vi "USB2CANFD_SchTest.vi"() -> ()   [LabVIEW 2010]
panel:
  in  "SpeedBpsDBT":u32(ring)=2000000 items=["5000 Kbps"=5000000, "2000 Kbps"=2000000, "1000 Kbps"=1000000, "500 Kbps"=500000, "250 Kbps"=250000, "200 Kbps"=200000, "125 Kbps"=125000, "100 Kbps"=100000, ""=0]
  in  "SpeedBpsNBT":u32(ring)=500000 items=["1000 Kbps"=1000000, "500 Kbps"=500000, "250 Kbps"=250000, "200 Kbps"=200000, "125 Kbps"=125000, "100 Kbps"=100000, ""=0]
  in  "TimePrecMs":u8=10
  in  "MsgTabIndex":u8
  in  "CanSendMsg7":T1={"ID"=7, "DLC"=8, "Flags"=0, "__Res0"=0, "__Res1"=0, "TimeStamp"=20, "Data[0]"=1, "Data[1]"=2, "Data[2]"=3, "Data[3]"=4, "Data[4]"=5, "Data[5]"=6, "Data[6]"=7, "Data[7]"=8, "Data[8]"=0, "Data[9]"=0, "Data[10]"=0, "Data[11]"=0, "Data[12]"=0, "Data[13]"=0, "Data[14]"=0, "Data[15]"=0, "Data[16]"=0, "Data[17]"=0, "Data[18]"=0, "Data[19]"=0, "Data[20]"=0, "Data[21]"=0, "Data[22]"=0, "Data[23]"=0, "Data[24]"=0, "Data[25]"=0, "Data[26]"=0, "Data[27]"=0, "Data[28]"=0, "Data[29]"=0, "Data[30]"=0, "Data[31]"=0, "Data[32]"=0, "Data[33]"=0, "Data[34]"=0, "Data[35]"=0, "Data[36]"=0, "Data[37]"=0, "Data[38]"=0, "Data[39]"=0, "Data[40]"=0, "Data[41]"=0, "Data[42]"=0, "Data[43]"=0, "Data[44]"=0, "Data[45]"=0, "Data[46]"=0, "Data[47]"=0, "Data[48]"=0, "Data[49]"=0, "Data[50]"=0, "Data[51]"=0, "Data[52]"=0, "Data[53]"=0, "Data[54]"=0, "Data[55]"=0, "Data[56]"=0, "Data[57]"=0, "Data[58]"=0, "Data[59]"=0, "Data[60]"=0, "Data[61]"=0, "Data[62]"=0, "Data[63]"=0} {"ID" format="%x"; "Data[1]" format="%x"; "Data[2]" format="%x"}
  in  "CanSendMsg6":T1={"ID"=6, "DLC"=8, "Flags"=0, "__Res0"=0, "__Res1"=0, "TimeStamp"=20, "Data[0]"=1, "Data[1]"=2, "Data[2]"=3, "Data[3]"=4, "Data[4]"=5, "Data[5]"=6, "Data[6]"=7, "Data[7]"=8, "Data[8]"=0, "Data[9]"=0, "Data[10]"=0, "Data[11]"=0, "Data[12]"=0, "Data[13]"=0, "Data[14]"=0, "Data[15]"=0, "Data[16]"=0, "Data[17]"=0, "Data[18]"=0, "Data[19]"=0, "Data[20]"=0, "Data[21]"=0, "Data[22]"=0, "Data[23]"=0, "Data[24]"=0, "Data[25]"=0, "Data[26]"=0, "Data[27]"=0, "Data[28]"=0, "Data[29]"=0, "Data[30]"=0, "Data[31]"=0, "Data[32]"=0, "Data[33]"=0, "Data[34]"=0, "Data[35]"=0, "Data[36]"=0, "Data[37]"=0, "Data[38]"=0, "Data[39]"=0, "Data[40]"=0, "Data[41]"=0, "Data[42]"=0, "Data[43]"=0, "Data[44]"=0, "Data[45]"=0, "Data[46]"=0, "Data[47]"=0, "Data[48]"=0, "Data[49]"=0, "Data[50]"=0, "Data[51]"=0, "Data[52]"=0, "Data[53]"=0, "Data[54]"=0, "Data[55]"=0, "Data[56]"=0, "Data[57]"=0, "Data[58]"=0, "Data[59]"=0, "Data[60]"=0, "Data[61]"=0, "Data[62]"=0, "Data[63]"=0} {"ID" format="%x"; "Data[1]" format="%x"; "Data[2]" format="%x"}
  in  "CanSendMsg5":T1={"ID"=5, "DLC"=8, "Flags"=0, "__Res0"=0, "__Res1"=0, "TimeStamp"=20, "Data[0]"=1, "Data[1]"=2, "Data[2]"=3, "Data[3]"=4, "Data[4]"=5, "Data[5]"=6, "Data[6]"=7, "Data[7]"=8, "Data[8]"=0, "Data[9]"=0, "Data[10]"=0, "Data[11]"=0, "Data[12]"=0, "Data[13]"=0, "Data[14]"=0, "Data[15]"=0, "Data[16]"=0, "Data[17]"=0, "Data[18]"=0, "Data[19]"=0, "Data[20]"=0, "Data[21]"=0, "Data[22]"=0, "Data[23]"=0, "Data[24]"=0, "Data[25]"=0, "Data[26]"=0, "Data[27]"=0, "Data[28]"=0, "Data[29]"=0, "Data[30]"=0, "Data[31]"=0, "Data[32]"=0, "Data[33]"=0, "Data[34]"=0, "Data[35]"=0, "Data[36]"=0, "Data[37]"=0, "Data[38]"=0, "Data[39]"=0, "Data[40]"=0, "Data[41]"=0, "Data[42]"=0, "Data[43]"=0, "Data[44]"=0, "Data[45]"=0, "Data[46]"=0, "Data[47]"=0, "Data[48]"=0, "Data[49]"=0, "Data[50]"=0, "Data[51]"=0, "Data[52]"=0, "Data[53]"=0, "Data[54]"=0, "Data[55]"=0, "Data[56]"=0, "Data[57]"=0, "Data[58]"=0, "Data[59]"=0, "Data[60]"=0, "Data[61]"=0, "Data[62]"=0, "Data[63]"=0} {"ID" format="%x"; "Data[1]" format="%x"; "Data[2]" format="%x"}
  in  "CanSendMsg4":T1={"ID"=4, "DLC"=8, "Flags"=0, "__Res0"=0, "__Res1"=0, "TimeStamp"=20, "Data[0]"=1, "Data[1]"=2, "Data[2]"=3, "Data[3]"=4, "Data[4]"=5, "Data[5]"=6, "Data[6]"=7, "Data[7]"=8, "Data[8]"=0, "Data[9]"=0, "Data[10]"=0, "Data[11]"=0, "Data[12]"=0, "Data[13]"=0, "Data[14]"=0, "Data[15]"=0, "Data[16]"=0, "Data[17]"=0, "Data[18]"=0, "Data[19]"=0, "Data[20]"=0, "Data[21]"=0, "Data[22]"=0, "Data[23]"=0, "Data[24]"=0, "Data[25]"=0, "Data[26]"=0, "Data[27]"=0, "Data[28]"=0, "Data[29]"=0, "Data[30]"=0, "Data[31]"=0, "Data[32]"=0, "Data[33]"=0, "Data[34]"=0, "Data[35]"=0, "Data[36]"=0, "Data[37]"=0, "Data[38]"=0, "Data[39]"=0, "Data[40]"=0, "Data[41]"=0, "Data[42]"=0, "Data[43]"=0, "Data[44]"=0, "Data[45]"=0, "Data[46]"=0, "Data[47]"=0, "Data[48]"=0, "Data[49]"=0, "Data[50]"=0, "Data[51]"=0, "Data[52]"=0, "Data[53]"=0, "Data[54]"=0, "Data[55]"=0, "Data[56]"=0, "Data[57]"=0, "Data[58]"=0, "Data[59]"=0, "Data[60]"=0, "Data[61]"=0, "Data[62]"=0, "Data[63]"=0} {"ID" format="%x"; "Data[1]" format="%x"; "Data[2]" format="%x"}
  in  "CanSendMsg3":T1={"ID"=3, "DLC"=8, "Flags"=0, "__Res0"=0, "__Res1"=0, "TimeStamp"=20, "Data[0]"=1, "Data[1]"=2, "Data[2]"=3, "Data[3]"=4, "Data[4]"=5, "Data[5]"=6, "Data[6]"=7, "Data[7]"=8, "Data[8]"=0, "Data[9]"=0, "Data[10]"=0, "Data[11]"=0, "Data[12]"=0, "Data[13]"=0, "Data[14]"=0, "Data[15]"=0, "Data[16]"=0, "Data[17]"=0, "Data[18]"=0, "Data[19]"=0, "Data[20]"=0, "Data[21]"=0, "Data[22]"=0, "Data[23]"=0, "Data[24]"=0, "Data[25]"=0, "Data[26]"=0, "Data[27]"=0, "Data[28]"=0, "Data[29]"=0, "Data[30]"=0, "Data[31]"=0, "Data[32]"=0, "Data[33]"=0, "Data[34]"=0, "Data[35]"=0, "Data[36]"=0, "Data[37]"=0, "Data[38]"=0, "Data[39]"=0, "Data[40]"=0, "Data[41]"=0, "Data[42]"=0, "Data[43]"=0, "Data[44]"=0, "Data[45]"=0, "Data[46]"=0, "Data[47]"=0, "Data[48]"=0, "Data[49]"=0, "Data[50]"=0, "Data[51]"=0, "Data[52]"=0, "Data[53]"=0, "Data[54]"=0, "Data[55]"=0, "Data[56]"=0, "Data[57]"=0, "Data[58]"=0, "Data[59]"=0, "Data[60]"=0, "Data[61]"=0, "Data[62]"=0, "Data[63]"=0} {"ID" format="%x"; "Data[1]" format="%x"; "Data[2]" format="%x"}
  in  "CanSendMsg2":T1={"ID"=2, "DLC"=8, "Flags"=0, "__Res0"=0, "__Res1"=0, "TimeStamp"=20, "Data[0]"=1, "Data[1]"=2, "Data[2]"=3, "Data[3]"=4, "Data[4]"=5, "Data[5]"=6, "Data[6]"=7, "Data[7]"=8, "Data[8]"=0, "Data[9]"=0, "Data[10]"=0, "Data[11]"=0, "Data[12]"=0, "Data[13]"=0, "Data[14]"=0, "Data[15]"=0, "Data[16]"=0, "Data[17]"=0, "Data[18]"=0, "Data[19]"=0, "Data[20]"=0, "Data[21]"=0, "Data[22]"=0, "Data[23]"=0, "Data[24]"=0, "Data[25]"=0, "Data[26]"=0, "Data[27]"=0, "Data[28]"=0, "Data[29]"=0, "Data[30]"=0, "Data[31]"=0, "Data[32]"=0, "Data[33]"=0, "Data[34]"=0, "Data[35]"=0, "Data[36]"=0, "Data[37]"=0, "Data[38]"=0, "Data[39]"=0, "Data[40]"=0, "Data[41]"=0, "Data[42]"=0, "Data[43]"=0, "Data[44]"=0, "Data[45]"=0, "Data[46]"=0, "Data[47]"=0, "Data[48]"=0, "Data[49]"=0, "Data[50]"=0, "Data[51]"=0, "Data[52]"=0, "Data[53]"=0, "Data[54]"=0, "Data[55]"=0, "Data[56]"=0, "Data[57]"=0, "Data[58]"=0, "Data[59]"=0, "Data[60]"=0, "Data[61]"=0, "Data[62]"=0, "Data[63]"=0} {"ID" format="%x"; "Data[1]" format="%x"; "Data[2]" format="%x"}
  in  "Receive Channel":u8(ring)=1 items=["CAN1", "CAN2"]
  out "Get Msg Num":i32
  out "pCanGetMsg OUT":T2(array[cluster])
  in  "stop":bool
  in  "CanSendMsg1":T1={"ID"=1, "DLC"=8, "Flags"=0, "__Res0"=0, "__Res1"=0, "TimeStamp"=20, "Data[0]"=1, "Data[1]"=2, "Data[2]"=3, "Data[3]"=4, "Data[4]"=5, "Data[5]"=6, "Data[6]"=7, "Data[7]"=8, "Data[8]"=0, "Data[9]"=0, "Data[10]"=0, "Data[11]"=0, "Data[12]"=0, "Data[13]"=0, "Data[14]"=0, "Data[15]"=0, "Data[16]"=0, "Data[17]"=0, "Data[18]"=0, "Data[19]"=0, "Data[20]"=0, "Data[21]"=0, "Data[22]"=0, "Data[23]"=0, "Data[24]"=0, "Data[25]"=0, "Data[26]"=0, "Data[27]"=0, "Data[28]"=0, "Data[29]"=0, "Data[30]"=0, "Data[31]"=0, "Data[32]"=0, "Data[33]"=0, "Data[34]"=0, "Data[35]"=0, "Data[36]"=0, "Data[37]"=0, "Data[38]"=0, "Data[39]"=0, "Data[40]"=0, "Data[41]"=0, "Data[42]"=0, "Data[43]"=0, "Data[44]"=0, "Data[45]"=0, "Data[46]"=0, "Data[47]"=0, "Data[48]"=0, "Data[49]"=0, "Data[50]"=0, "Data[51]"=0, "Data[52]"=0, "Data[53]"=0, "Data[54]"=0, "Data[55]"=0, "Data[56]"=0, "Data[57]"=0, "Data[58]"=0, "Data[59]"=0, "Data[60]"=0, "Data[61]"=0, "Data[62]"=0, "Data[63]"=0} {"ID" format="%x"; "Data[1]" format="%x"; "Data[2]" format="%x"}
  in  "Send Channel":u8(ring) items=["CAN1", "CAN2"]
  in  "Device Index":i32(ring) items=["0", "1", "2", "3", "4", "5"]
  in  "pCanGetMsg":T1
  in  "pCanConfig":T3={"Mode"=0, "ISOCRCEnable"=1, "RetrySend"=1, "ResEnable"=1, "NBT_BRP"=1, "NBT_SEG1"=59, "NBT_SEG2"=20, "NBT_SJW"=2, "DBT_BRP"=1, "DBT_SEG1"=14, "DBT_SEG2"=5, "DBT_SJW"=2, "__Res0[0]"=0, "__Res0[1]"=0, "__Res0[2]"=0, "__Res0[3]"=0, "__Res0[4]"=0, "__Res0[5]"=0, "__Res0[6]"=0, "__Res0[7]"=0}
  # "测试之前将CAN1和CAN2对接，也就是CAN1的H接CAN2的H，CAN1的L接CAN2的L，CAN1调度表模式发送数据，CAN2接收数据"
  # "MsgTabIndex为0时发送前3帧，为1时发送后4帧"
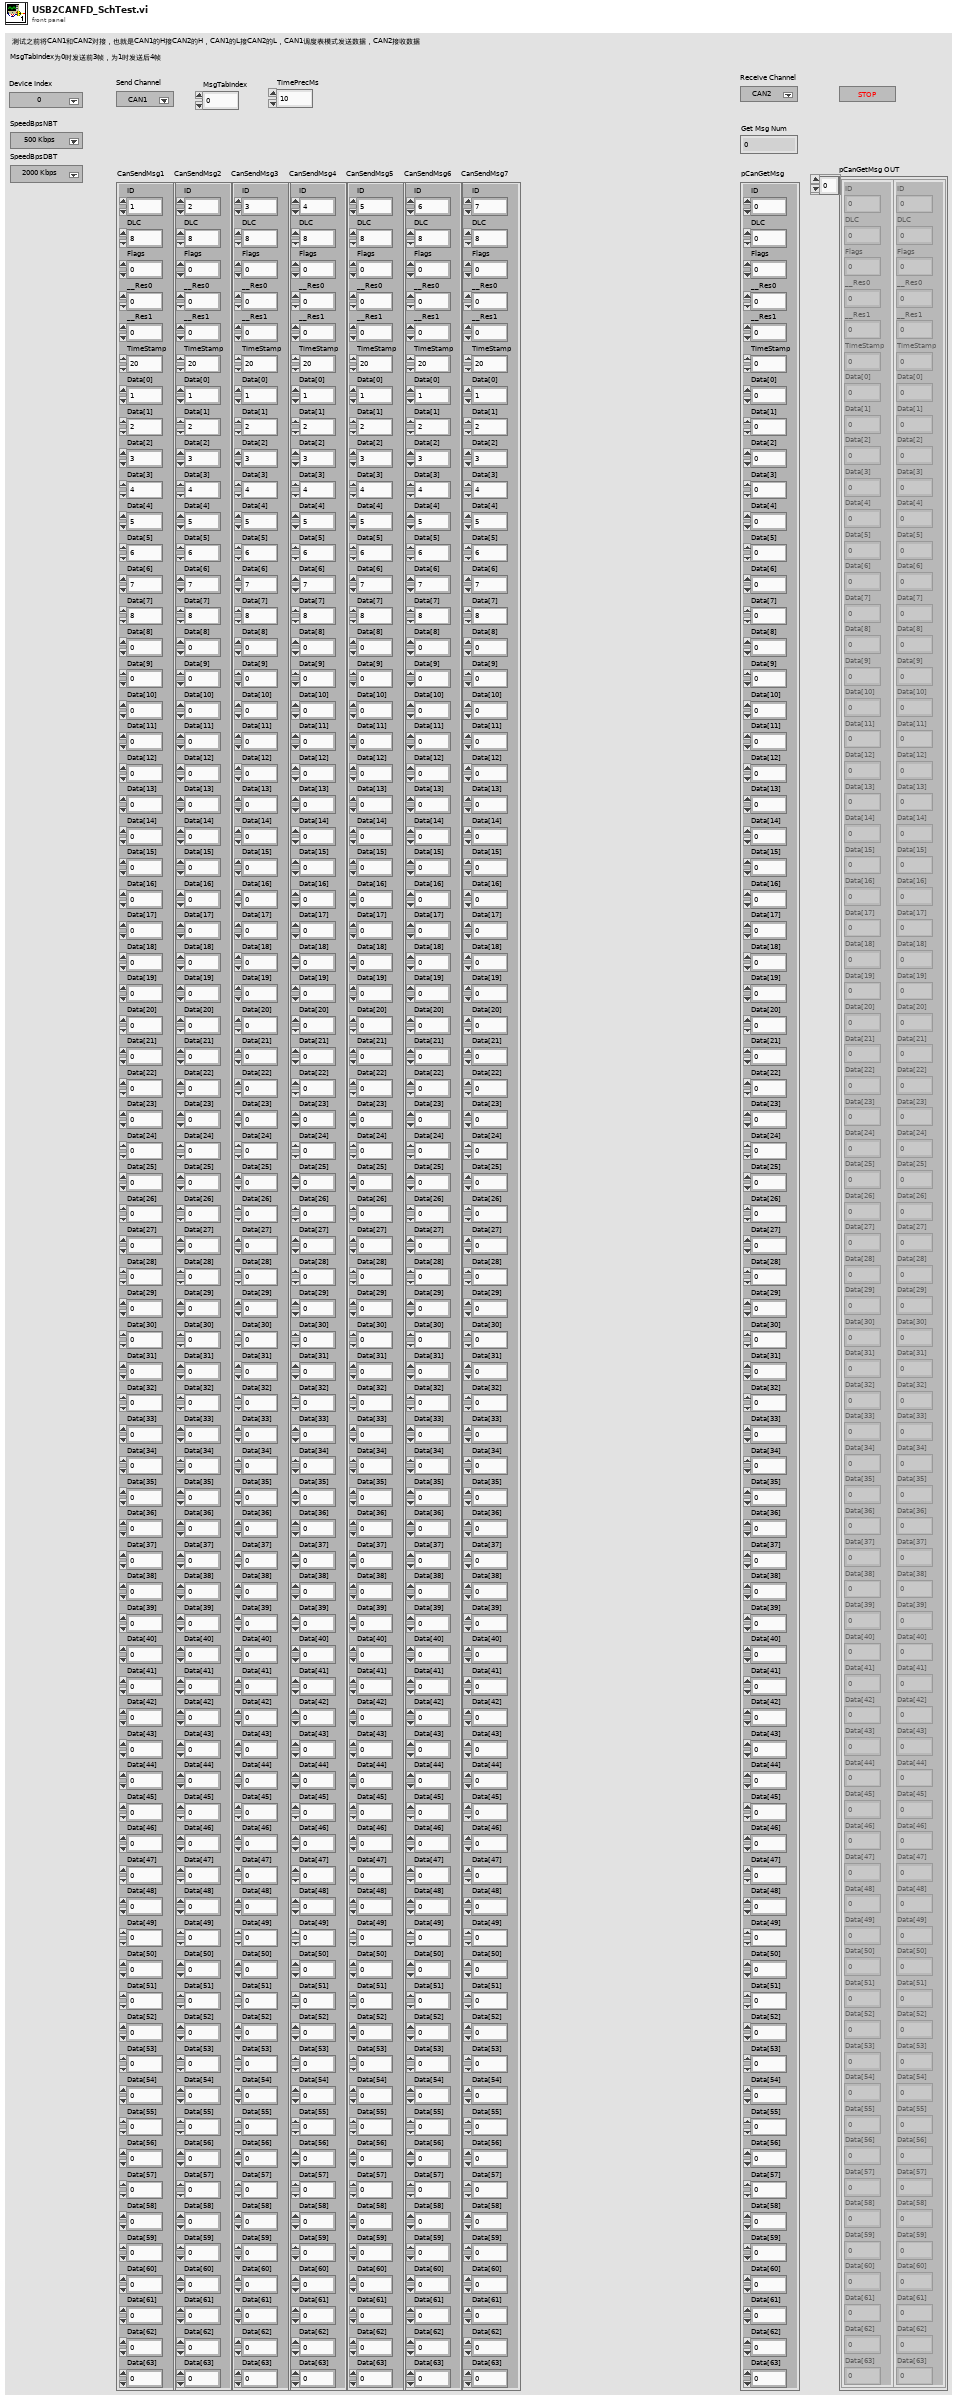
[diagram p1: front panel]
types:
  T1 = cluster{"ID":u32, "DLC":u8, "Flags":u8, "__Res0":u8, "__Res1":u8, "TimeStamp":u32, "Data[0]":u8, "Data[1]":u8, "Data[2]":u8, "Data[3]":u8, "Data[4]":u8, "Data[5]":u8, "Data[6]":u8, "Data[7]":u8, "Data[8]":u8, "Data[9]":u8, "Data[10]":u8, "Data[11]":u8, "Data[12]":u8, "Data[13]":u8, "Data[14]":u8, "Data[15]":u8, "Data[16]":u8, "Data[17]":u8, "Data[18]":u8, "Data[19]":u8, "Data[20]":u8, "Data[21]":u8, "Data[22]":u8, "Data[23]":u8, "Data[24]":u8, "Data[25]":u8, "Data[26]":u8, "Data[27]":u8, "Data[28]":u8, "Data[29]":u8, "Data[30]":u8, "Data[31]":u8, "Data[32]":u8, "Data[33]":u8, "Data[34]":u8, "Data[35]":u8, "Data[36]":u8, "Data[37]":u8, "Data[38]":u8, "Data[39]":u8, "Data[40]":u8, "Data[41]":u8, "Data[42]":u8, "Data[43]":u8, "Data[44]":u8, "Data[45]":u8, "Data[46]":u8, "Data[47]":u8, "Data[48]":u8, "Data[49]":u8, "Data[50]":u8, "Data[51]":u8, "Data[52]":u8, "Data[53]":u8, "Data[54]":u8, "Data[55]":u8, "Data[56]":u8, "Data[57]":u8, "Data[58]":u8, "Data[59]":u8, "Data[60]":u8, "Data[61]":u8, "Data[62]":u8, "Data[63]":u8}
  T2 = cluster{"ID":u32, "DLC":u8, "Flags":u8, "__Res0":u8, "__Res1":u8, "TimeStamp":u32, "Data[0]":u8, "Data[1]":u8, "Data[2]":u8, "Data[3]":u8, "Data[4]":u8, "Data[5]":u8, "Data[6]":u8, "Data[7]":u8, "Data[8]":u8, "Data[9]":u8, "Data[10]":u8, "Data[11]":u8, "Data[12]":u8, "Data[13]":u8, "Data[14]":u8, "Data[15]":u8, "Data[16]":u8, "Data[17]":u8, "Data[18]":u8, "Data[19]":u8, "Data[20]":u8, "Data[21]":u8, "Data[22]":u8, "Data[23]":u8, "Data[24]":u8, "Data[25]":u8, "Data[26]":u8, "Data[27]":u8, "Data[28]":u8, "Data[29]":u8, "Data[30]":u8, "Data[31]":u8, "Data[32]":u8, "Data[33]":u8, "Data[34]":u8, "Data[35]":u8, "Data[36]":u8, "Data[37]":u8, "Data[38]":u8, "Data[39]":u8, "Data[40]":u8, "Data[41]":u8, "Data[42]":u8, "Data[43]":u8, "Data[44]":u8, "Data[45]":u8, "Data[46]":u8, "Data[47]":u8, "Data[48]":u8, "Data[49]":u8, "Data[50]":u8, "Data[51]":u8, "Data[52]":u8, "Data[53]":u8, "Data[54]":u8, "Data[55]":u8, "Data[56]":u8, "Data[57]":u8, "Data[58]":u8, "Data[59]":u8, "Data[60]":u8, "Data[61]":u8, "Data[62]":u8, "Data[63]":u8}[]
  T3 = cluster{"Mode":u8, "ISOCRCEnable":u8, "RetrySend":u8, "ResEnable":u8, "NBT_BRP":u8, "NBT_SEG1":u8, "NBT_SEG2":u8, "NBT_SJW":u8, "DBT_BRP":u8, "DBT_SEG1":u8, "DBT_SEG2":u8, "DBT_SJW":u8, "__Res0[0]":u8, "__Res0[1]":u8, "__Res0[2]":u8, "__Res0[3]":u8, "__Res0[4]":u8, "__Res0[5]":u8, "__Res0[6]":u8, "__Res0[7]":u8}
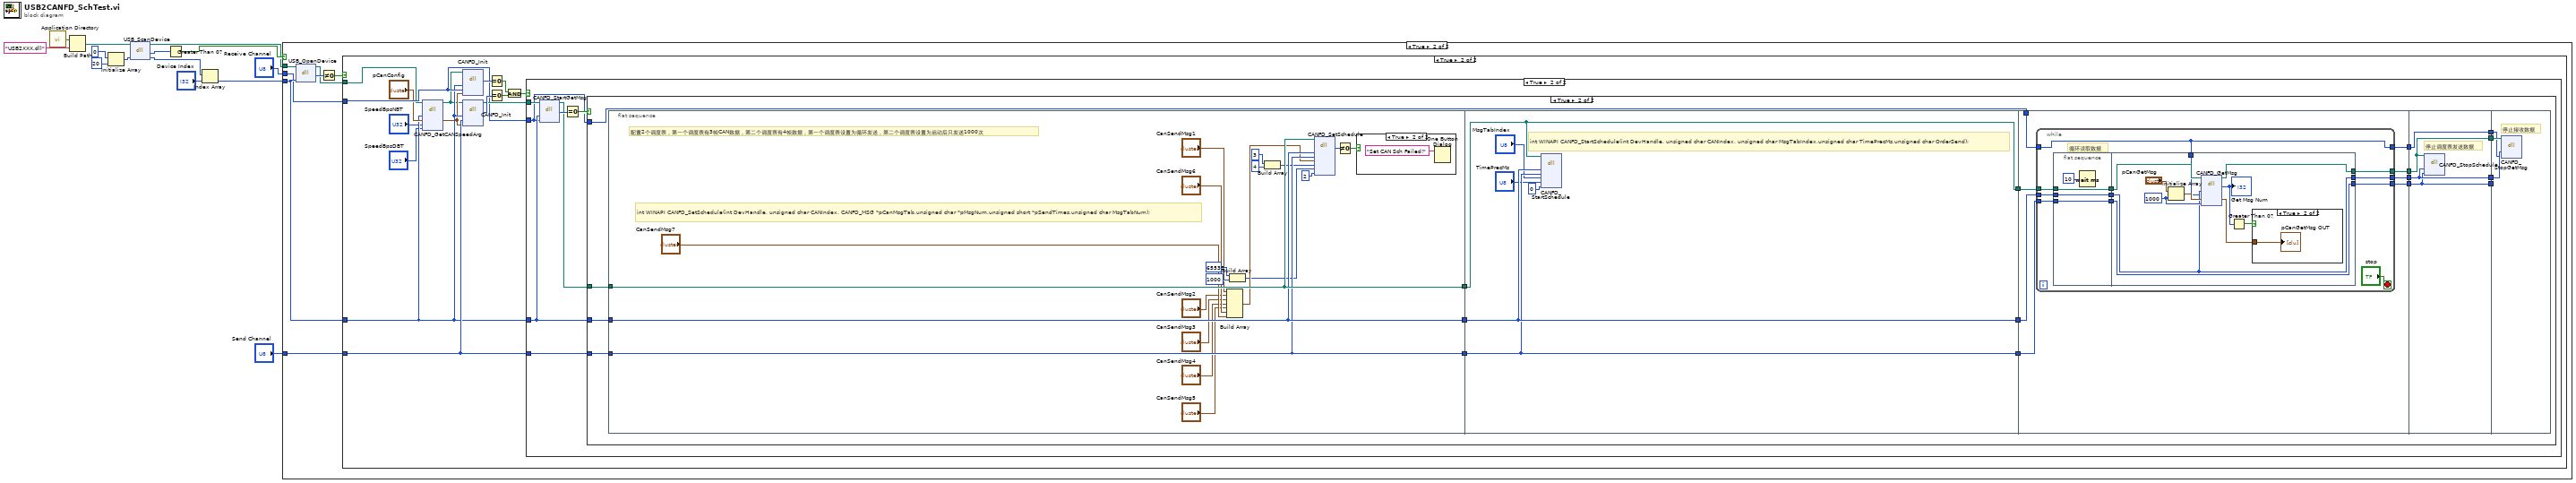
[diagram p0: block diagram]
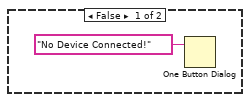
[diagram p2: hidden frame]
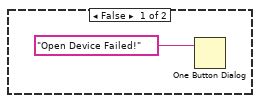
[diagram p3: hidden frame]
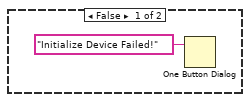
[diagram p4: hidden frame]
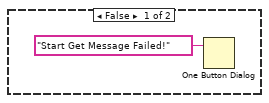
[diagram p5: hidden frame]
diagram:
  n1 = call <vilib>:"Application Directory.vi"() -> ("Application Directory"=w2:path)
  n2 = Build Path(base path=w2, name or relative path="USB2XXX.dll") -> (appended path=w1:path)
  n3 = Initialize Array(0, 20 ("dimension size")) -> (w14:i32[])
  n4 = dll-call lib="E:/OtherWork/STM32/USB2XXX_Example/sdk/api/Labview/USB2XXX.dll" fn="USB_ScanDevice"(path in=w1, "pDevNum"=w14) -> (path out=w5:path, "return type"=w10:i32, "pDevNum"=w11:i32[])  [unwired: 2 in, 1 out]
  n5 = Greater Than 0?(x=w10) -> (x > 0?=w9:bool)
  n6 = Index Array(array=w11, index="Device Index") -> (element=w7:i32)
  n7 = case shown="True" w9 {
    tunnel: w7 -> [_ w19]
    tunnel: w5 -> [_ w20]
    tunnel: "Send Channel" -> [_ w18]
    tunnel: "Receive Channel" -> [_ w16]
    frame False {
      n8 = One Button Dialog(message="No Device Connected!") -> ()  [unwired: 1 in, 1 out]
    }
    frame True {
      n9 = dll-call lib="E:/OtherWork/STM32/USB2XXX_Example/sdk/api/Labview/USB2XXX.*" fn="USB_OpenDevice"(path in=w20, "DevHandle"=w19) -> (path out=w17:path, "return type"=w22:u8)  [unwired: 3 in, 1 out]
      n10 = Not Equal To 0?(x=w22) -> (x != 0?=w21:bool)
      n11 = case shown="True" w21 {
        tunnel: w17 -> [_ w25]
        tunnel: w19 -> [_ w29]
        tunnel: w18 -> [_ w36]
        tunnel: w16 -> [_ w31]
        frame False {
          n12 = One Button Dialog(message="Open Device Failed!") -> ()  [unwired: 1 in, 1 out]
        }
        frame True {
          n13 = dll-call lib="E:/Projects/USB2XXX/trunk/USB2XXX/USB2XXX/vs2019/Release/USB2XXX.*" fn="CANFD_GetCANSpeedArg"(path in=w25, "DevHandle"=w29, "pCanConfig"="pCanConfig", "SpeedBpsNBT"="SpeedBpsNBT", "SpeedBpsDBT"="SpeedBpsDBT") -> (path out=w24:path, "pCanConfig"=w26:T3)  [unwired: 6 in, 1 out]
          n14 = dll-call lib="E:/OtherWork/STM32/USB2XXX_Example/sdk/api/Labview/USB2XXX.*" fn="CANFD_Init"(path in=w24, "DevHandle"=w29, "CANIndex"=w31, "pCanConfig"=w26) -> ("return type"=w35:i32)  [unwired: 5 in, 2 out]
          n15 = dll-call lib="E:/OtherWork/STM32/USB2XXX_Example/sdk/api/Labview/USB2XXX.*" fn="CANFD_Init"(path in=w24, "DevHandle"=w29, "CANIndex"=w36, "pCanConfig"=w26) -> (path out=w37:path, "return type"=w38:i32)  [unwired: 5 in, 1 out]
          n16 = Equal To 0?(x=w35) -> (x = 0?=w34:bool)
          n17 = Equal To 0?(x=w38) -> (x = 0?=w33:bool)
          n18 = And(x=w34, y=w33) -> (x .and. y?=w32:bool)
          n19 = case shown="True" w32 {
            tunnel: w37 -> [_ w46]
            tunnel: w29 -> [_ w41]
            tunnel: w36 -> [_ w42]
            tunnel: w31 -> [_ w40]
            frame False {
              n20 = One Button Dialog(message="Initialize Device Failed!") -> ()  [unwired: 1 in, 1 out]
            }
            frame True {
              n21 = dll-call lib="E:/OtherWork/STM32/USB2XXX_Example/sdk/api/Labview/USB2XXX.*" fn="CANFD_StartGetMsg"(path in=w46, "DevHandle"=w41, "CANIndex"=w40) -> (path out=w43:path, "return type"=w45:i32)  [unwired: 4 in, 1 out]
              n22 = Equal To 0?(x=w45) -> (x = 0?=w44:bool)
              n23 = case shown="True" w44 {
                tunnel: w43 -> [_ w65]
                tunnel: w42 -> [_ w64]
                tunnel: w41 -> [_ w63]
                tunnel: w40 -> [_ w56]
                frame False {
                  n24 = One Button Dialog(message="Start Get Message Failed!") -> ()  [unwired: 1 in, 1 out]
                }
                frame True {
                  n25 = flat-sequence {
                    tunnel: w63 -> [w84]
                    tunnel: w64 -> [w83]
                    tunnel: w65 -> [w85]
                    tunnel: [w85] -> w53
                    tunnel: [w83] -> w51
                    tunnel: [w84] -> w49
                    tunnel: w53 -> [w92]
                    tunnel: [w92] -> w52
                    tunnel: w51 -> [w90]
                    tunnel: [w90] -> w50
                    tunnel: w49 -> [w91]
                    tunnel: [w91] -> w48
                    tunnel: [w97] -> w62
                    tunnel: [w96] -> w60
                    tunnel: [w95] -> w58
                    tunnel: w52 -> [w100]
                    tunnel: w50 -> [w99]
                    tunnel: w48 -> [w98]
                    tunnel: w56 -> [w94]
                    tunnel: [w93] -> w55
                    tunnel: w62 -> [w131]
                    tunnel: [w131] -> w61
                    tunnel: w60 -> [w130]
                    tunnel: [w130] -> w59
                    tunnel: w58 -> [w129]
                    tunnel: [w129] -> w57
                    tunnel: w55 -> [w128]
                    tunnel: [w128] -> w54
                    tunnel: w61 -> [w134]
                    tunnel: w59 -> [w133]
                    tunnel: w57 -> [_]
                    tunnel: w54 -> [w132]
                    frame #0 {
                      # "配置2个调度表，第一个调度表有3帧CAN数据，第二个调度表有4帧数据，第一个调度表设置为循环发送，第二个调度表设置为启动后只发送1000次"
                      # "int WINAPI CANFD_SetSchedule(int DevHandle, unsigned char CANIndex, CANFD_MSG *pCanMsgTab,unsigned char *pMsgNum,unsigned short *pSendTimes,unsigned char MsgTabNum);"
                      n26 = Build Array("CanSendMsg1", "CanSendMsg2", "CanSendMsg3", "CanSendMsg4", "CanSendMsg5", "CanSendMsg6", "CanSendMsg7") -> (w76:T2)
                      n27 = Build Array(u16 65535 ("element"), u16 1000 ("element")) -> (w70:u16[])
                      n28 = Build Array(u8 3 ("element"), u8 4 ("element")) -> (w71:u8[])
                      n29 = dll-call lib="E:/Projects/USB2XXX/trunk/USB2XXX/USB2XXX/vs2010/Release/USB2XXX.*" fn="CANFD_SetSchedule"(path in=w85, "DevHandle"=w84, "CANIndex"=w83, "pCanMsgTab"=w76, "pMsgNum"=w71, "pSendTimes"=w70, "MsgTabNum"=u8 2) -> ("return type"=w67:i32)  [unwired: 8 in, 2 out]
                      n30 = Not Equal To 0?(x=w67) -> (x != 0?=w68:bool)
                      n31 = case shown="True" w68 {
                        frame False {
                        }
                        frame True {
                          n32 = One Button Dialog(message="Set CAN Sch Failed!") -> ()  [unwired: 1 in, 1 out]
                        }
                      }
                    }
                    frame #1 {
                      # "int WINAPI CANFD_StartSchedule(int DevHandle, unsigned char CANIndex, unsigned char MsgTabIndex,unsigned char TimePrecMs,unsigned char OrderSend);"
                      n33 = dll-call lib="E:/Projects/USB2XXX/trunk/USB2XXX/USB2XXX/vs2010/Release/USB2XXX.*" fn="CANFD_StartSchedule"(path in=w92, "DevHandle"=w91, "CANIndex"=w90, "MsgTabIndex"="MsgTabIndex", "TimePrecMs"="TimePrecMs", "OrderSend"=u8 0) -> ()  [unwired: 8 in, 2 out]
                    }
                    frame #2 {
                      n34 = while {
                        tunnel: w100 -> [w104]
                        tunnel: w99 -> [w105]
                        tunnel: w98 -> [w103]
                        tunnel: [w102] -> w97
                        tunnel: [w107] -> w96
                        tunnel: [w106] -> w95
                        tunnel: w94 -> [w101]
                        tunnel: [w101] -> w93
                        stop <- "stop" stop-if-true
                        # "循环读取数据"
                        n35 = flat-sequence {
                          tunnel: [w114] -> w110
                          tunnel: [w112] -> w109
                          tunnel: [w113] -> w108
                          tunnel: w105 -> [w114]
                          tunnel: w104 -> [w113]
                          tunnel: w103 -> [w112]
                          tunnel: w110 -> [w119]
                          tunnel: w109 -> [w121]
                          tunnel: w108 -> [w123]
                          tunnel: [w121] -> w107
                          tunnel: [w119] -> w106
                          tunnel: [w120] -> w102
                          tunnel: w101 -> [w118]
                          frame #0 {
                            n36 = Wait (ms)(milliseconds to wait=u32 10 ("等待时间（毫秒）")) -> ()  [unwired: 1 out]
                          }
                          frame #1 {
                            w124 = 1000 ("BufferSize")
                            n37 = Initialize Array("pCanGetMsg", w124) -> (w125:T2)
                            n38 = dll-call lib="E:/OtherWork/STM32/USB2XXX_Example/sdk/api/Labview/USB2XXX.dll" fn="CANFD_GetMsg"(path in=w123, "DevHandle"=w121, "CANIndex"=w118, "pCanGetMsg"=w125, "BufferSize"=w124) -> (path out=w120:path, "return type"=w117:i32, "pCanGetMsg"=w122:T2)  [unwired: 5 in, 1 out]
                            "Get Msg Num" <- w117
                            n39 = Greater Than 0?(x=w117) -> (x > 0?=w116:bool)
                            n40 = case shown="True" w116 {
                              tunnel: w122 -> [_ w127]
                              frame False {
                              }
                              frame True {
                                "pCanGetMsg OUT" <- w127
                              }
                            }
                          }
                        }
                      }
                    }
                    frame #3 {
                      # "停止调度表发送数据"
                      n41 = dll-call lib="E:/Projects/USB2XXX/trunk/USB2XXX/USB2XXX/vs2010/Release/USB2XXX.*" fn="CANFD_StopSchedule"(path in=w131, "DevHandle"=w130, "CANIndex"=w129) -> ()  [unwired: 5 in, 2 out]
                    }
                    frame #4 {
                      # "停止接收数据"
                      n42 = dll-call lib="E:/OtherWork/STM32/USB2XXX_Example/sdk/api/Labview/USB2XXX.*" fn="CANFD_StopGetMsg"(path in=w134, "DevHandle"=w133, "CANIndex"=w132) -> ()  [unwired: 5 in, 2 out]
                    }
                  }
                }
              }
            }
          }
        }
      }
    }
  }
